vi "FarfiledDefineReferencePose.vi"(2 "当前位置":i32, 3 "参考位置集合":cluster{"数组":i32[], "数组":i32[]}) -> (0 "未执行位置":cluster{"数组":i32[], "数组":i32[]}, 1 "已经执行位置":cluster{"数组":i32[], "数组":i32[]})   [LabVIEW 2018]
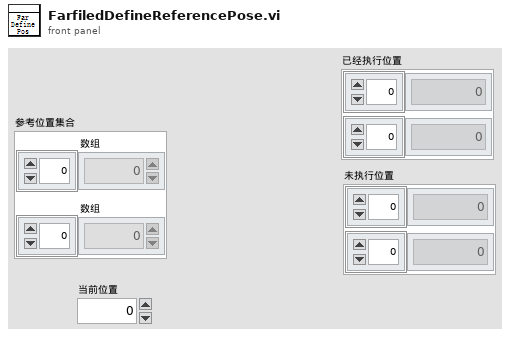
[diagram p1: front panel]
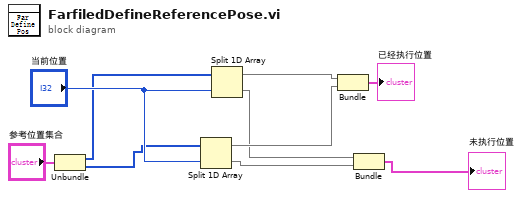
[diagram p0: block diagram]
diagram:
  n1 = Unbundle("参考位置集合") -> ("数组"=w2:i32[], "数组"=w1:i32[])
  n2 = Split 1D Array(array=w1, index="当前位置") -> (first subarray=w7:i32[], second subarray=w5:i32[])
  n3 = Split 1D Array(array=w2, index="当前位置") -> (first subarray=w8:i32[], second subarray=w6:i32[])
  n4 = Bundle(w8, w7) -> (→"已经执行位置":cluster{i32[], i32[]})  [unwired: 1 in]
  n5 = Bundle(w6, w5) -> (→"未执行位置":cluster{i32[], i32[]})  [unwired: 1 in]
